vi "加表当量解析.vi"(11 "输入":i32) -> (2 "x/y":sgl, 3 "输出":string)   [LabVIEW 2012]
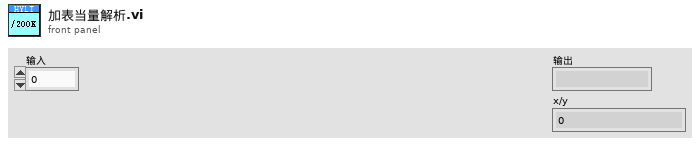
[diagram p1: front panel]
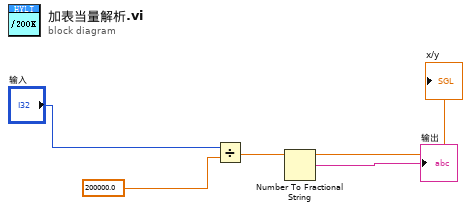
[diagram p0: block diagram]
diagram:
  n1 = Divide(x="输入", y=sgl 200000.0) -> (x/y=w2:sgl)
  "x/y" <- w2
  n2 = Number To Fractional String(number=w2) -> (F-format string=→"输出":string)  [unwired: 3 in]
